vi "Dimming Command.vi"(8 "error in (no error)":errorcluster, 10 "Dimming value":u16, 11 "Lutron QS Object in":refnum<class "Lutron QS Object.lvclass">) -> (0 "error out":errorcluster, 3 "Lutron QS Object out":refnum<class "Lutron QS Object.lvclass">)   [LabVIEW 2016, in "Lutron QS Control Protocol.lvlib" / "Lutron QS Object.lvclass"]
uses:
  Lutron QS Object.lvclass
  Labview Tool box/String Contains.vi
panel:
  out "VISA resource name out":refnum<visa-resource-name>
  out "concatenated string":string
  out "Array 2":i32[](array[numeric])
  out "Array":string[](array[string])
  out "return count":u32
  out "read buffer":string
  out "length":i32
  out "Numeric Control":i32
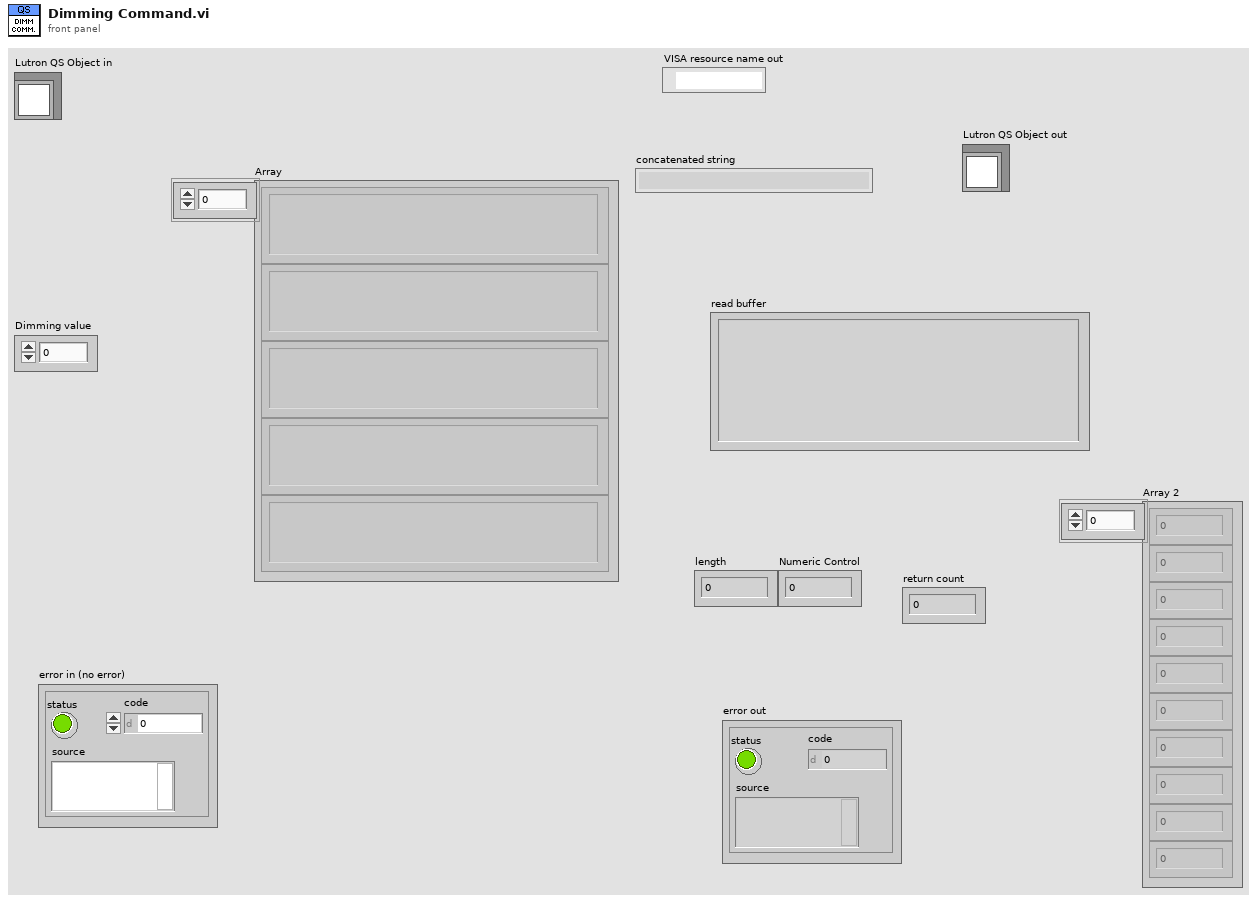
[diagram p1: front panel]
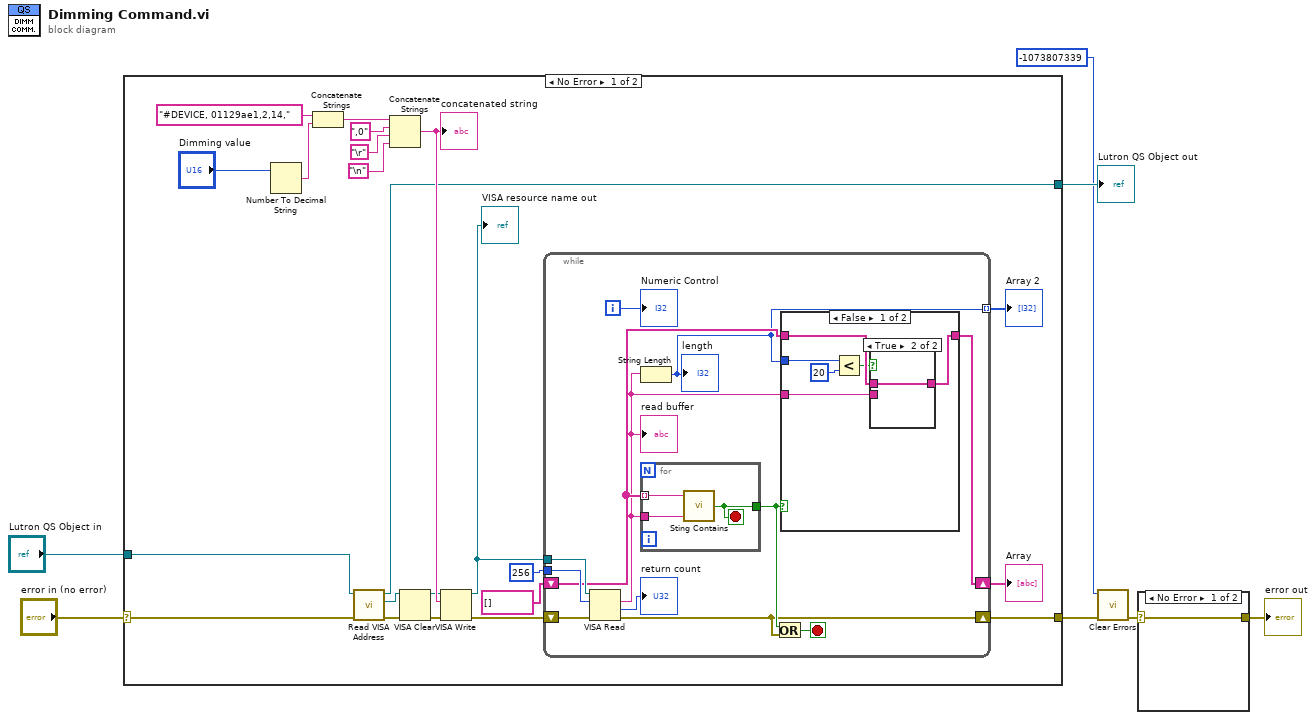
[diagram p0: block diagram]
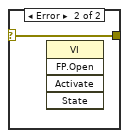
[diagram p2: hidden frame]
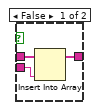
[diagram p3: hidden frame]
diagram:
  n1 = case shown="No Error" "error in (no error)" {
    selector: "error in (no error)" -> [w12 w57]
    tunnel: [w15 w57] -> w2
    tunnel: [w13 w56] -> w5
    tunnel: "Lutron QS Object in" -> [w14 w56]
    frame No Error {
      n2 = Number To Decimal String(number="Dimming value") -> (decimal integer string=w28:string)  [unwired: 1 in]
      n3 = Concatenate Strings("#DEVICE, 01129ae1,2,14," ("Dimming Command"), w28) -> (w17:string)
      n4 = call-dynamic "Read VISA Address.vi"("error in (no error)"=w12, "Generic Device in"=w14) -> ("error out"=w10:errorcluster, "VISA Address"=w11:refnum<visa-resource-name>, "Generic Device out"=w13:refnum<class "Lutron QS Object.lvclass">)  [unwired: 7 in]
      n5 = Concatenate Strings(w17, ",0" ("string"), "\r", "\n") -> (w18:string)
      "concatenated string" <- w18
      n6 = VISA Clear(VISA resource name=w11, error in (no error)=w10) -> (VISA resource name out=w9:refnum<visa-resource-name>, error out=w8:errorcluster)
      n7 = VISA Write(VISA resource name=w9, write buffer=w18, error in (no error)=w8) -> (VISA resource name out=w24:refnum<visa-resource-name>, error out=w23:errorcluster)  [unwired: 1 out]
      "VISA resource name out" <- w24
      n8 = while {
        tunnel: w24 -> [w41]
        shift-right: [w32] -> w15
        shift-left: w23 -> [w40]
        tunnel: u32 256 ("byte count") -> [w37]
        shift-right: [w34] -> w19
        shift-left: string[] [] -> [w36]
        tunnel: [w30] -> w20 mode=indexing
        i -> [w38]
        stop <- w31 stop-if-true
        n9 = VISA Read(VISA resource name=w41, byte count=w37, error in (no error)=w40) -> (read buffer=w35:string, return count=→"return count":u32, error out=w32:errorcluster)  [unwired: 1 out]
        "read buffer" <- w35
        n10 = String Length(string=w35) -> (length=w30:i32)
        "length" <- w30
        n11 = for {
          tunnel: [w55] -> w33
          tunnel: w36 -> [w54] mode=indexing
          tunnel: w35 -> [w53]
          stop <- w55 stop-if-true
          n12 = call "Sting Contains.vi"("Regular expression"=w53, "Input String"=w54) -> ("Found?"=w55:bool)  [unwired: 2 in, 1 out]
        }
        n13 = Or(x=w33, y=w32) -> (x .or. y?=w31:bool)
        n14 = case shown="False" w33 {
          tunnel: w36 -> [w47 w52]
          tunnel: w35 -> [w46 _]
          tunnel: [w45 w52] -> w34
          tunnel: w30 -> [w44 _]
          frame False {
            n15 = Less?(x=w44, y=20) -> (x < y?=w42:bool)
            n16 = case shown="True" w42 {
              tunnel: w47 -> [w50 w51]
              tunnel: w46 -> [w49 _]
              tunnel: [w48 w51] -> w45
              frame False {
                n17 = Insert Into Array(array=w50, new element=w49) -> (w48:string[])  [unwired: 1 in]
              }
              frame True {
              }
            }
          }
          frame True {
          }
        }
        "Numeric Control" <- w38
      }
      "Array" <- w19
      "Array 2" <- w20
    }
    frame Error {
    }
  }
  "Lutron QS Object out" <- w5
  n18 = call <vilib>:"Clear Errors.vi"("error in (no error)"=w2, "specific error code to clear (0: all)"=-1073807339) -> ("error out"=w1:errorcluster)  [unwired: 4 in, 1 out]
  n19 = case shown="No Error" w1 {
    selector: w1 -> [w58 w59]
    tunnel: [w58 w59] -> w4
    frame No Error {
    }
    frame Error {
      n20 = invoke class="VI" method="FP.Open"() -> ()  [unwired: 5 in, 5 out]
    }
  }
  "error out" <- w4
